vi "Test Time Measurement.vi"() -> (0 "VI Tester Testing time (seconds)":dbl, 1 "Caraya Testing time (seconds)":dbl, 2 "ICov Testing time (seconds)":dbl, 3 "UTF Testing time (seconds)":dbl)   [LabVIEW 2018]
uses:
  <vilib>/utf/common/utf_test_result.ctl
  Caraya Time Measurement.vi
  <vilib>/utf/NI_UnitTestFramework.lvlib
panel:
  out "No. of Tests":i32=10
  in  "Multiplier of runs":i32=10
  in  "Action Update Set Point":bool=TRUE
  in  "Action Update Ramp Rate":bool=TRUE
  in  "Action Update Heater State":bool=TRUE
  in  "All Test":bool
  out "Caraya report":string
  out "Caraya In Progress":bool
  out "VI Tester report":string
  out "VI Tester In Progress":bool
  out "ICov Results":enum16{"PASSED", "FAILED", "ERROR"}[](array[ring])
  out "ICov In Progress":bool
  out "UTF In Progress":bool
  out "UTF Results":T1[](array[typedef])
  # "If this button checked, then other buttons are ignored."
  # "UTF"
  # "VI Tester"
  # "ICov"
  # "Caraya"
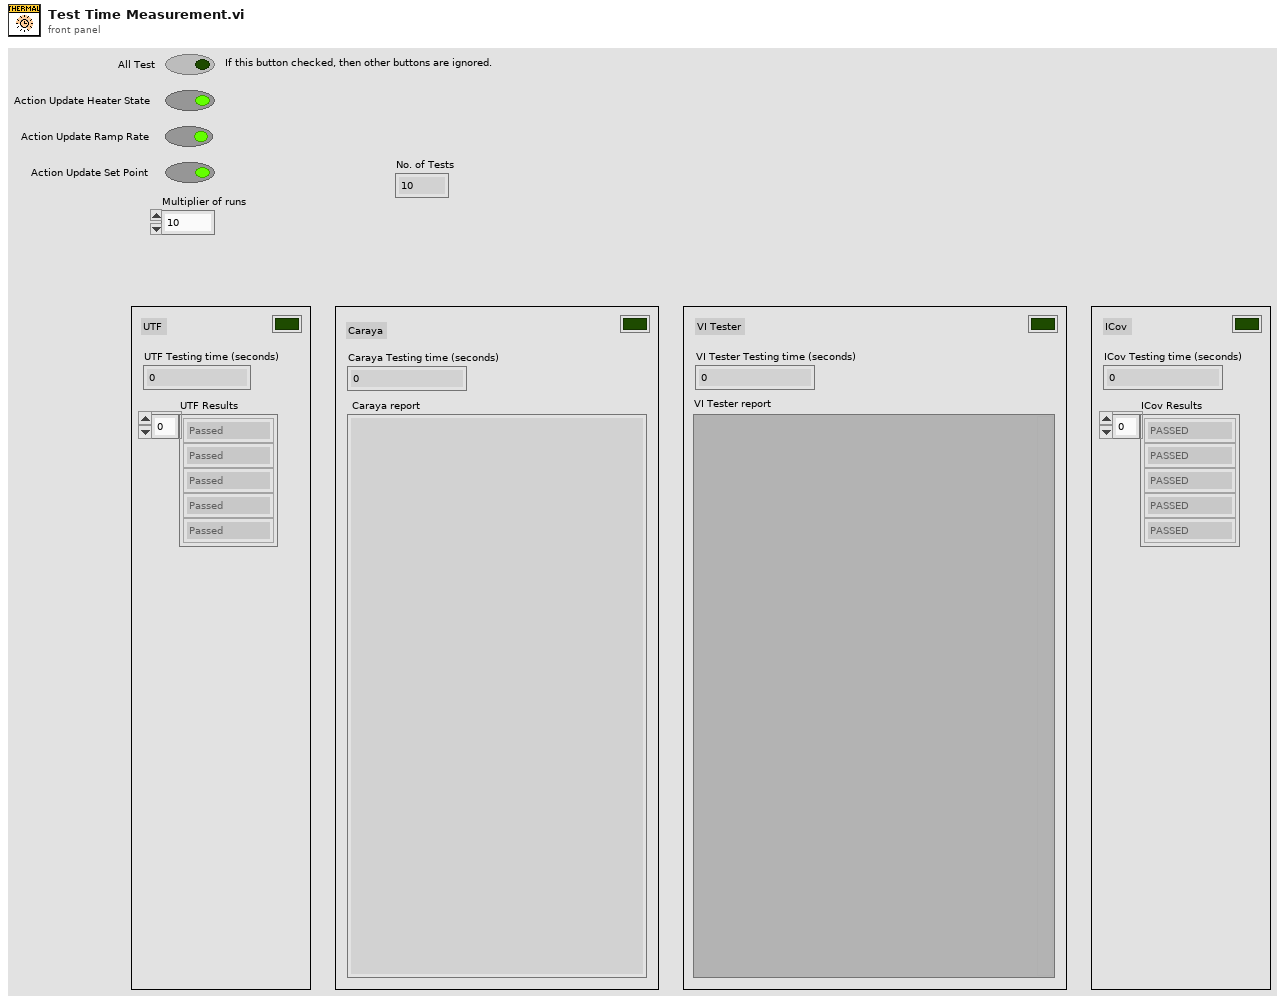
[diagram p1: front panel]
types:
  T1 = typedef "NI_UnitTestFramework.lvlib/utf_test_result.ctl" = enum16{"Passed", "Failed", "Error", "Skipped", "Not Processed"}
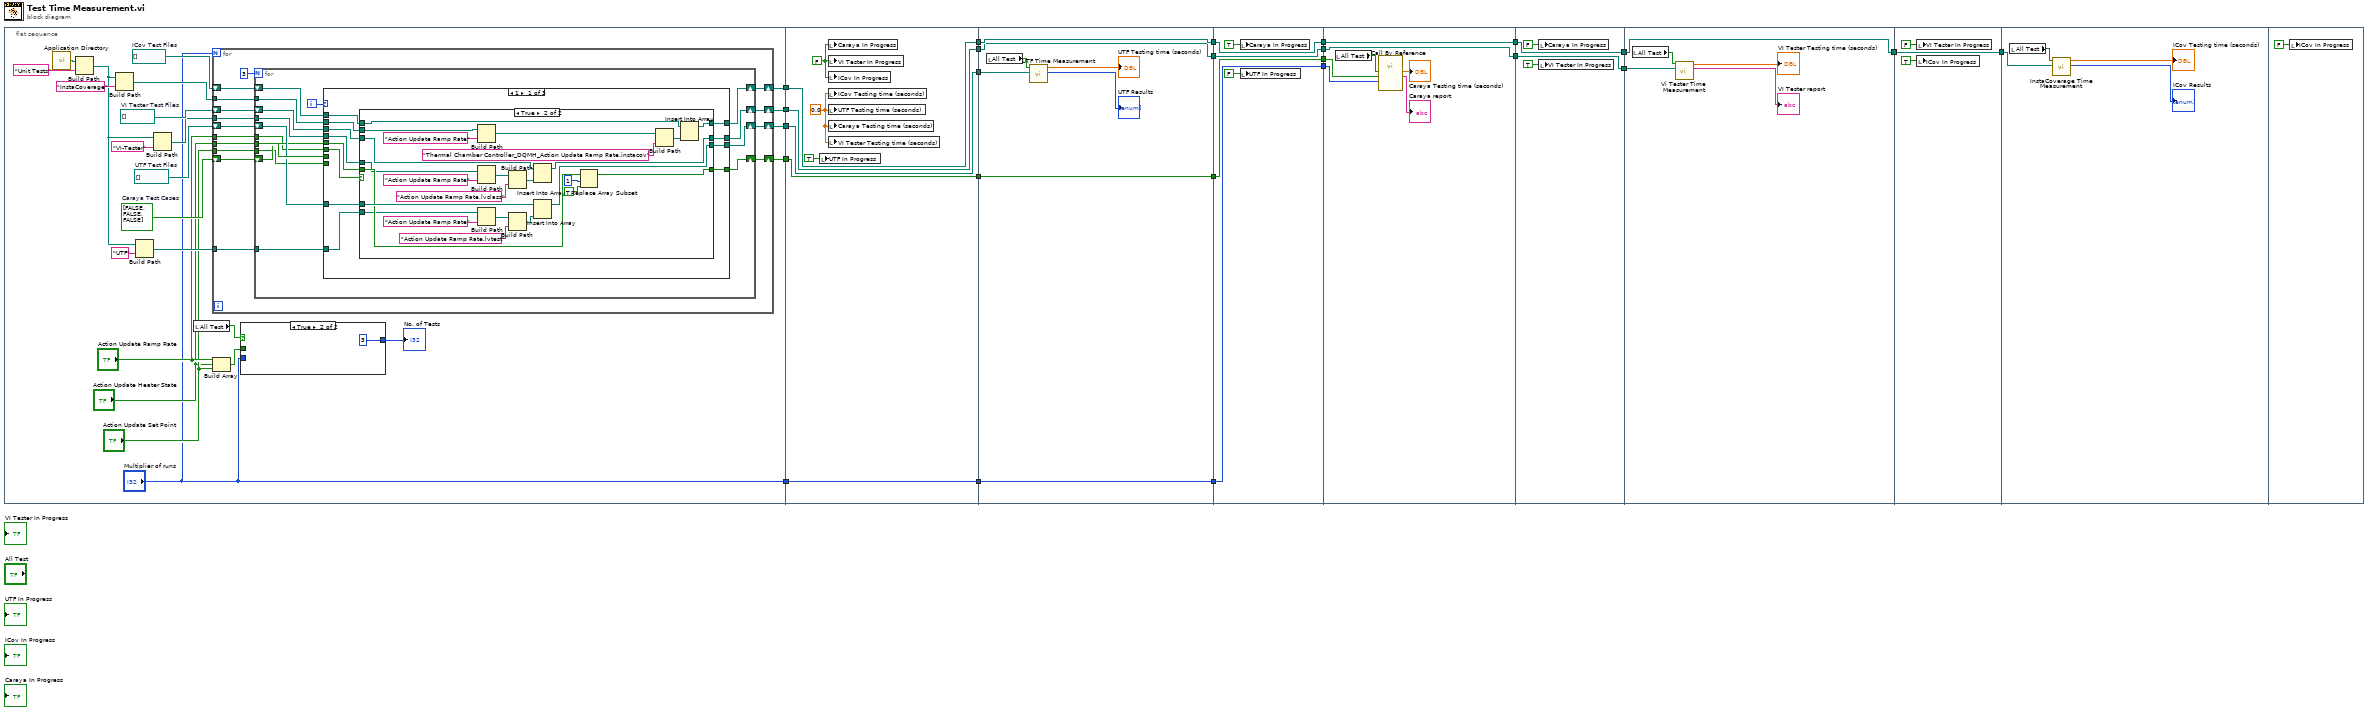
[diagram p0: block diagram]
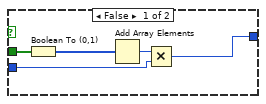
[diagram p2: hidden frame]
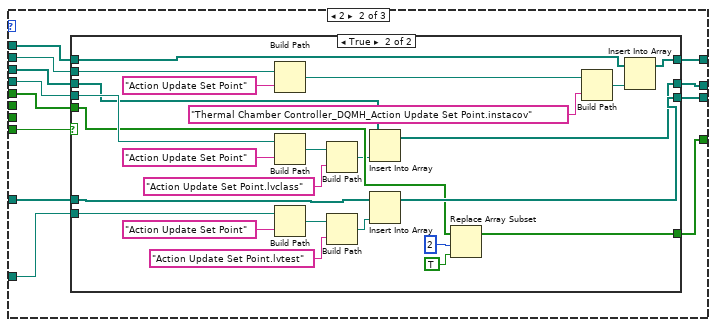
[diagram p4: hidden frame]
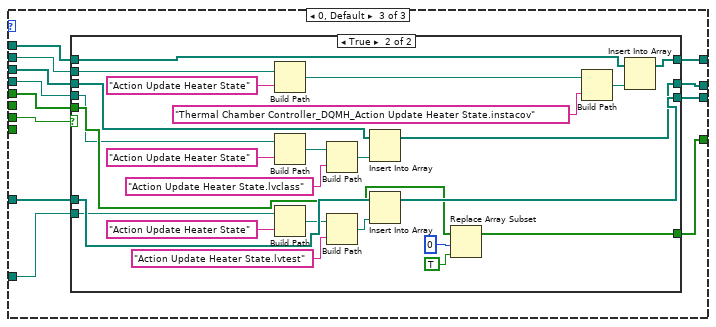
[diagram p6: hidden frame]
diagram:
  n1 = flat-sequence {
    tunnel: [w36] -> w24
    tunnel: [w35] -> w15
    tunnel: [w34] -> w9
    tunnel: [w33] -> w8
    tunnel: ["Multiplier of runs"] -> w4
    tunnel: w24 -> [w212]
    tunnel: [w212] -> w23
    tunnel: [w211] -> w16
    tunnel: w15 -> [w211]
    tunnel: [w210] -> w10
    tunnel: w9 -> [w210]
    tunnel: w8 -> [w209]
    tunnel: [w209] -> w7
    tunnel: w4 -> [w208]
    tunnel: [w208] -> w3
    tunnel: w23 -> [w220]
    tunnel: [w219] -> w17
    tunnel: w16 -> [w219]
    tunnel: [w218] -> w11
    tunnel: w10 -> [w218]
    tunnel: w7 -> [w217]
    tunnel: [w217] -> w6
    tunnel: w3 -> [w216]
    tunnel: [w216] -> w2
    tunnel: [w227] -> w18
    tunnel: w17 -> [w227]
    tunnel: [w226] -> w12
    tunnel: w11 -> [w226]
    tunnel: w6 -> [w225]
    tunnel: [w225] -> w5
    tunnel: w2 -> [w224]
    tunnel: [w224] -> w1
    tunnel: [w233] -> w19
    tunnel: w18 -> [w233]
    tunnel: [w232] -> w13
    tunnel: w12 -> [w232]
    tunnel: w5 -> [w231]
    tunnel: w1 -> [w230]
    tunnel: [w238] -> w20
    tunnel: w19 -> [w238]
    tunnel: [w237] -> w14
    tunnel: w13 -> [w237]
    tunnel: [w242] -> w21
    tunnel: w20 -> [w242]
    tunnel: w14 -> [w241]
    tunnel: [w246] -> w22
    tunnel: w21 -> [w246]
    tunnel: w22 -> [w249]
    frame #0 {
      w41 = path[] []  # ICov Test Files
      w46 = path[] []  # VI Tester Test Files
      w47 = bool[] [FALSE, FALSE, FALSE]  # Caraya Test Cases
      w48 = path[] []  # UTF Test Files
      n2 = call <vilib>:"Application Directory.vi"() -> ("Application Directory"=w45:path)
      n3 = Build Path(base path=w45, name or relative path="Unit Tests") -> (appended path=w39:path)
      n4 = Build Path(base path=w39, name or relative path="InstaCoverage") -> (appended path=w37:path)
      n5 = Build Path(base path=w39, name or relative path="UTF") -> (appended path=w38:path)
      n6 = Build Path(base path=w39, name or relative path="VI-Tester") -> (appended path=w32:path)
      n7 = local read "All Test"() -> (w31:bool)
      n8 = for {
        N: "Multiplier of runs" -> [_]
        tunnel: "Action Update Heater State" -> [w69]
        tunnel: w38 -> [w64]
        tunnel: w37 -> [w63]
        tunnel: "Action Update Ramp Rate" -> [w62]
        tunnel: "Action Update Set Point" -> [w61]
        tunnel: w32 -> [w56]
        shift-right: [w59] -> w35
        shift-left: w41 -> [w65]
        shift-right: [w58] -> w34
        shift-left: w46 -> [w66]
        shift-right: [w60] -> w36
        shift-left: w48 -> [w68]
        shift-right: [w57] -> w33
        shift-left: w47 -> [w67]
        n9 = for {
          N: 3 -> [_]
          tunnel: w69 -> [w84]
          tunnel: w64 -> [w75]
          tunnel: w63 -> [w74]
          tunnel: w56 -> [w73]
          shift-right: [w78] -> w60
          shift-left: w68 -> [w83]
          shift-right: [w79] -> w58
          shift-left: w66 -> [w81]
          shift-right: [w76] -> w59
          shift-left: w65 -> [w80]
          shift-right: [w77] -> w57
          shift-left: w67 -> [w82]
          tunnel: w62 -> [w71]
          tunnel: w61 -> [w70]
          i -> [w72]
          n10 = case shown="1" w72 {
            tunnel: w84 -> [_ _ w178]
            tunnel: w83 -> [w96 w136 w177]
            tunnel: w82 -> [w90 w130 w176]
            tunnel: w81 -> [w94 w134 w175]
            tunnel: w80 -> [w92 w132 w174]
            tunnel: [w88 w128 w173] -> w79
            tunnel: [w89 w129 w172] -> w78
            tunnel: [w86 w126 w171] -> w77
            tunnel: [w87 w127 w170] -> w76
            tunnel: w75 -> [w95 w135 w169]
            tunnel: w74 -> [w91 w131 w168]
            tunnel: w73 -> [w93 w133 w167]
            tunnel: w71 -> [w85 _ _]
            tunnel: w70 -> [_ w137 _]
            frame 1 {
              n11 = case shown="True" w85 {
                tunnel: w96 -> [w100 w125]
                tunnel: [w100 w124] -> w89
                tunnel: w90 -> [w99 w123]
                tunnel: [w99 w120] -> w86
                tunnel: w94 -> [w98 w119]
                tunnel: [w98 w118] -> w88
                tunnel: w95 -> [_ w116]
                tunnel: w92 -> [w97 w112]
                tunnel: [w97 w111] -> w87
                tunnel: w91 -> [_ w109]
                tunnel: w93 -> [_ w107]
                frame False {
                }
                frame True {
                  n12 = Build Path(base path=w109, name or relative path="Action Update Ramp Rate") -> (appended path=w105:path)
                  n13 = Build Path(base path=w107, name or relative path="Action Update Ramp Rate") -> (appended path=w102:path)
                  n14 = Build Path(base path=w116, name or relative path="Action Update Ramp Rate") -> (appended path=w115:path)
                  n15 = Build Path(base path=w102, name or relative path="Action Update Ramp Rate.lvclass") -> (appended path=w101:path)
                  n16 = Build Path(base path=w115, name or relative path="Action Update Ramp Rate.lvtest") -> (appended path=w113:path)
                  n17 = Insert Into Array(array=w119, new element=w101) -> (w118:path[])  [unwired: 1 in]
                  n18 = Insert Into Array(array=w125, new element=w113) -> (w124:path[])  [unwired: 1 in]
                  n19 = Replace Array Subset(array=w123, new element=TRUE, index=1) -> (w120:bool[])
                  n20 = Build Path(base path=w105, name or relative path="Thermal Chamber Controller_DQMH_Action Update Ramp Rate.instacov") -> (appended path=w104:path)
                  n21 = Insert Into Array(array=w112, new element=w104) -> (w111:path[])  [unwired: 1 in]
                }
              }
            }
            frame 2 {
              n22 = case shown="True" w137 {
                tunnel: [w141 w166] -> w129
                tunnel: [w138 w163] -> w126
                tunnel: [w140 w162] -> w128
                tunnel: w135 -> [_ w160]
                tunnel: [w139 w156] -> w127
                tunnel: w131 -> [_ w154]
                tunnel: w133 -> [_ w152]
                tunnel: w136 -> [w141 w148]
                tunnel: w134 -> [w140 w147]
                tunnel: w132 -> [w139 w146]
                tunnel: w130 -> [w138 w145]
                frame False {
                }
                frame True {
                  n23 = Build Path(base path=w154, name or relative path="Action Update Set Point") -> (appended path=w150:path)
                  n24 = Build Path(base path=w152, name or relative path="Action Update Set Point") -> (appended path=w143:path)
                  n25 = Build Path(base path=w160, name or relative path="Action Update Set Point") -> (appended path=w159:path)
                  n26 = Build Path(base path=w143, name or relative path="Action Update Set Point.lvclass") -> (appended path=w142:path)
                  n27 = Build Path(base path=w159, name or relative path="Action Update Set Point.lvtest") -> (appended path=w157:path)
                  n28 = Insert Into Array(array=w147, new element=w142) -> (w162:path[])  [unwired: 1 in]
                  n29 = Insert Into Array(array=w148, new element=w157) -> (w166:path[])  [unwired: 1 in]
                  n30 = Replace Array Subset(array=w145, new element=TRUE, index=2) -> (w163:bool[])
                  n31 = Build Path(base path=w150, name or relative path="Thermal Chamber Controller_DQMH_Action Update Set Point.instacov") -> (appended path=w149:path)
                  n32 = Insert Into Array(array=w146, new element=w149) -> (w156:path[])  [unwired: 1 in]
                }
              }
            }
            frame 0, Default {
              n33 = case shown="True" w178 {
                tunnel: w177 -> [w182 w207]
                tunnel: [w182 w206] -> w172
                tunnel: w176 -> [w181 w205]
                tunnel: [w181 w202] -> w171
                tunnel: w175 -> [w180 w201]
                tunnel: [w180 w200] -> w173
                tunnel: w169 -> [_ w198]
                tunnel: w174 -> [w179 w194]
                tunnel: [w179 w193] -> w170
                tunnel: w168 -> [_ w191]
                tunnel: w167 -> [_ w189]
                frame False {
                }
                frame True {
                  n34 = Build Path(base path=w191, name or relative path="Action Update Heater State") -> (appended path=w187:path)
                  n35 = Build Path(base path=w189, name or relative path="Action Update Heater State") -> (appended path=w184:path)
                  n36 = Build Path(base path=w198, name or relative path="Action Update Heater State") -> (appended path=w197:path)
                  n37 = Build Path(base path=w184, name or relative path="Action Update Heater State.lvclass") -> (appended path=w185:path)
                  n38 = Build Path(base path=w197, name or relative path="Action Update Heater State.lvtest") -> (appended path=w195:path)
                  n39 = Insert Into Array(array=w201, new element=w185) -> (w200:path[])  [unwired: 1 in]
                  n40 = Insert Into Array(array=w207, new element=w195) -> (w206:path[])  [unwired: 1 in]
                  n41 = Replace Array Subset(array=w205, new element=TRUE, index=0) -> (w202:bool[])
                  n42 = Build Path(base path=w187, name or relative path="Thermal Chamber Controller_DQMH_Action Update Heater State.instacov") -> (appended path=w186:path)
                  n43 = Insert Into Array(array=w194, new element=w186) -> (w193:path[])  [unwired: 1 in]
                }
              }
            }
          }
        }
      }
      n44 = Build Array("Action Update Ramp Rate", "Action Update Heater State", "Action Update Set Point") -> (w30:bool[])
      n45 = case shown="True" w31 {
        tunnel: w30 -> [w53 _]
        tunnel: "Multiplier of runs" -> [w51 _]
        tunnel: [w49 3 ("Multiplier of runs")] -> w25
        frame False {
          n46 = Boolean To (0,1)(Boolean=w53) -> (0, 1=w52:i16[])
          n47 = Add Array Elements(numeric array=w52) -> (sum=w50:i16)
          n48 = Multiply(x=w50, y=w51) -> (x*y=w49:i32)
        }
        frame True {
        }
      }
      "No. of Tests" <- w25
    }
    frame #1 {
      w214 = FALSE
      w213 = 0.0
      n49 = local write "UTF In Progress"(TRUE) -> ()
      n50 = local write "Caraya In Progress"(w214) -> ()
      n51 = local write "VI Tester In Progress"(w214) -> ()
      n52 = local write "ICov In Progress"(w214) -> ()
      n53 = local write "ICov Testing time (seconds)"(w213) -> ()
      n54 = local write "UTF Testing time (seconds)"(w213) -> ()
      n55 = local write "Caraya Testing time (seconds)"(w213) -> ()
      n56 = local write "VI Tester Testing time (seconds)"(w213) -> ()
    }
    frame #2 {
      n57 = local read "All Test"() -> (w221:bool)
      n58 = call "UTF Time Measurement.vi"("test file paths"=w220, "All Test"=w221) -> ("UTF Results"=→"UTF Results":T1[], "UTF Testing time (seconds)"=→"UTF Testing time (seconds)":dbl)  [unwired: 8 in]
    }
    frame #3 {
      n59 = local write "Caraya In Progress"(TRUE) -> ()
      n60 = local write "UTF In Progress"(FALSE) -> ()
    }
    frame #4 {
      n61 = local read "All Test"() -> (w234:bool)
      n62 = call-by-ref "Call By Reference"("No. of Runs"=w230, "Test Cases"=w231, "All Test"=w234) -> ("Caraya report"=→"Caraya report":string, "ICov Testing time (seconds)"=→"Caraya Testing time (seconds)":dbl)  [unwired: 9 in, 2 out]
    }
    frame #5 {
      n63 = local write "Caraya In Progress"(FALSE) -> ()
      n64 = local write "VI Tester In Progress"(TRUE) -> ()
    }
    frame #6 {
      n65 = local read "All Test"() -> (w243:bool)
      n66 = call "Vi Tester Time Measurement.vi"("test file paths"=w241, "All Test"=w243) -> ("VI Tester report"=→"VI Tester report":string, "VI Tester Testing time (seconds)"=→"VI Tester Testing time (seconds)":dbl)  [unwired: 8 in]
    }
    frame #7 {
      n67 = local write "VI Tester In Progress"(FALSE ("ICov In Progress")) -> ()
      n68 = local write "ICov In Progress"(TRUE ("ICov In Progress")) -> ()
    }
    frame #8 {
      n69 = local read "All Test"() -> (w250:bool)
      n70 = call "InstaCoverage Time Measurement.vi"("test file paths"=w249, "All Test"=w250) -> ("ICov Results"=→"ICov Results":enum16{"PASSED", "FAILED", "ERROR"}[], "ICov Testing time (seconds)"=→"ICov Testing time (seconds)":dbl)  [unwired: 8 in]
    }
    frame #9 {
      n71 = local write "ICov In Progress"(FALSE ("ICov In Progress")) -> ()
    }
  }
